vi "Update test_serialize_deserialize Bundle.vi"(8 "error in (no error)":errorcluster, 11 "Diagram in":refnum<vi>) -> (0 "error out":errorcluster, 3 "Diagram out":refnum<vi>)   [LabVIEW 2020]
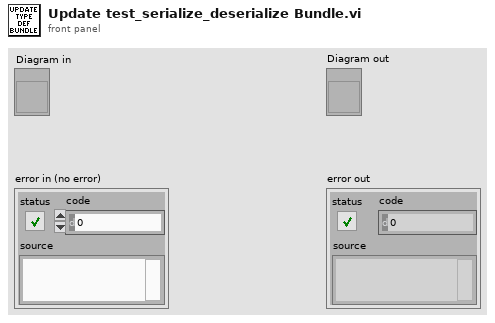
[diagram p1: front panel]
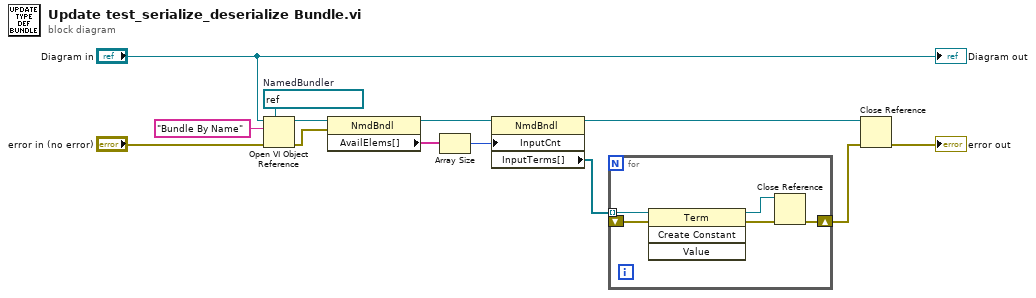
[diagram p0: block diagram]
diagram:
  w8 = refnum<vi> refnum  # NamedBundler
  n1 = Open VI Object Reference(7:w8, 8:"error in (no error)", 10:"Bundle By Name" ("name/order"), 11:"Diagram in") -> (0:w13:errorcluster, 3:w12:refnum<vi>)
  n2 = property class="NmdBndl"(reference=w12, error in=w13) -> (reference out=w5:refnum<vi>, "AvailElems[]"=w6:string[])  [unwired: 1 out]
  n3 = Array Size(array=w6) -> (size(s)=w7:i32)
  n4 = property class="NmdBndl"(reference=w5, "InputCnt"=w7) -> (reference out=w11:refnum<vi>, "InputTerms[]"=w9:refnum<vi>[])  [unwired: 1 in, 1 out]
  n5 = for {
    tunnel: w9 -> [w18] mode=indexing
    shift-right: [w15] -> w10
    shift-left: _ -> [w14]
    n6 = invoke class="Term" method="Create Constant"(reference=w18, error in=w14) -> (reference out=w17:refnum<vi>, error out=w16:errorcluster)  [unwired: 2 in, 2 out]
    n7 = Close Reference(reference=w17, error in (no error)=w16) -> (error out=w15:errorcluster)
  }
  n8 = Close Reference(reference=w11, error in (no error)=w10) -> (error out=→"error out":errorcluster)
  "Diagram out" <- "Diagram in"
